vi "ToTable.vi"(8 "error in":errorcluster, 9 "Table Index (0)":i32, 10 "variant":variant, 11 "Benchmark PID editor node in":refnum<class "Benchmark PID editor node.lvclass">) -> (0 "error out":errorcluster, 1 "row headers":string[](array[string]), 2 "table":string[][](array[string]), 3 "Benchmark PID editor node out":refnum<class "Benchmark PID editor node.lvclass">)   [LabVIEW 2018, in "Benchmark PID editor node.lvclass"]
doc: "Generates the strings needed to display on a table based on the information found in the engine and module configuration classes."
uses:
  Benchmark PID editor node.lvclass
  module/configuration/Benchmark PID configuration.lvclass
  <vilib>/NI/Tag Bus/tag/tag descriptor.lvclass
  <vilib>/NI/Module Execution Interface/Engine Configuration/engine configuration.lvclass
  <vilib>/NI/Configuration Framework/serializable configuration/NISE_CEF_serializable configuration.lvclass
  C:/Program Files (x86)/National Instruments/LabVIEW 2018/vi.lib/NI/Tag Bus Module Framework/module configuration/TBM module configuration.lvclass
  C:/Program Files (x86)/National Instruments/LabVIEW 2018/vi.lib/NI/Tag Bus Module Framework/root configuration/TBM configuration.lvclass
  C:/Program Files (x86)/National Instruments/LabVIEW 2018/vi.lib/NI/Configuration Framework/serializable configuration/NISE_CEF_serializable configuration.lvclass
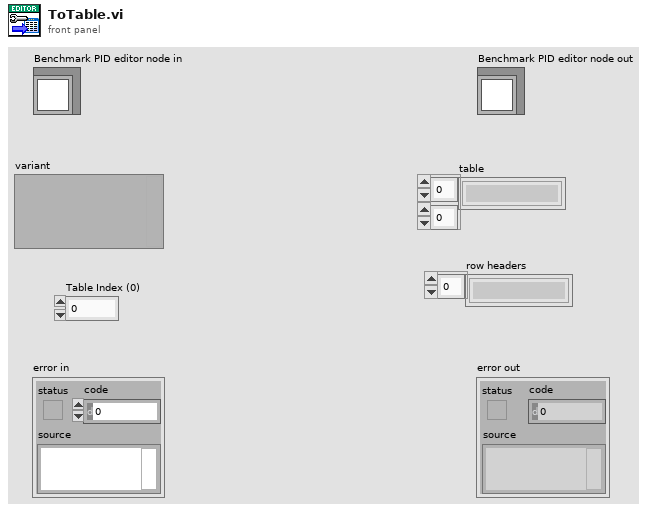
[diagram p1: front panel]
types:
  T1 = typedef "Benchmark PID configuration.lvclass/Line.ctl" = cluster{"PID Name":string, "Setpoint":refnum<class "TBM channel.lvclass">, "Variable":refnum<class "TBM channel.lvclass">, "Output":refnum<class "TBM channel.lvclass">}
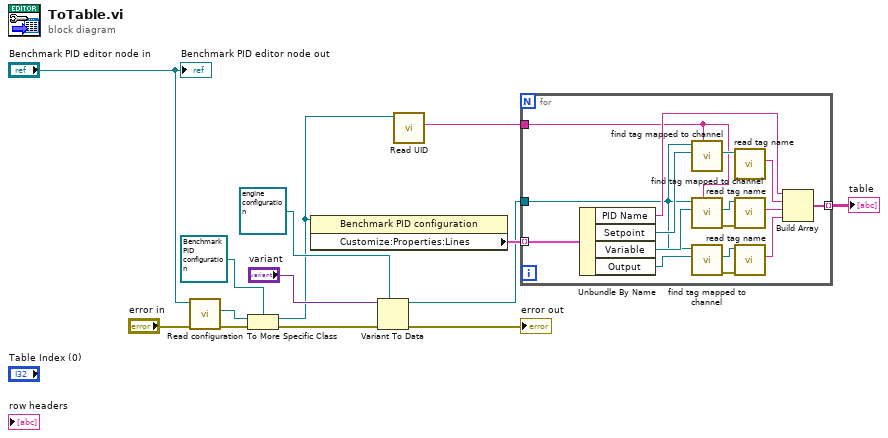
[diagram p0: block diagram]
diagram:
  n1 = call-dynamic "Read configuration.vi"("error in"="error in", "Benchmark PID editor node in"="Benchmark PID editor node in") -> ("error out"=w14:errorcluster, "configuration"=w5:refnum<class "NISE_CEF_serializable configuration.lvclass">)  [unwired: 7 in, 1 out]
  n2 = To More Specific Class(target class=refnum<class "Benchmark PID configuration.lvclass"> refnum ("tag bus configurable plugin module configuration"), reference=w5, error in=w14) -> (specific class reference=w4:refnum<class "Benchmark PID configuration.lvclass">, error out=w2:errorcluster)
  n3 = property class="Benchmark PID configuration"(reference=w4) -> ("Customize:Properties:Lines"=w11:T1[])  [unwired: 1 in, 2 out]
  n4 = Variant To Data(error in=w2, type=refnum<class "engine configuration.lvclass"> refnum ("engine configuration"), Variant="variant") -> (data=w8:refnum<class "engine configuration.lvclass">, error out=→"error out":errorcluster)
  n5 = call <vilib>:"Read UID.vi"("configuration in"=w4) -> ("instance id"=w3:string)  [unwired: 8 in, 2 out]
  n6 = for {
    tunnel: w11 -> [w30] mode=indexing
    tunnel: w8 -> [w17]
    tunnel: [w26] -> w6 mode=indexing
    tunnel: w3 -> [w21]
    n7 = Unbundle By Name(w30) -> ("PID Name"=w25:string, "Setpoint"=w27:refnum<class "TBM channel.lvclass">, "Variable"=w20:refnum<class "TBM channel.lvclass">, "Output"=w18:refnum<class "TBM channel.lvclass">)
    n8 = call <vilib>:"find tag mapped to channel.vi"("owner"=w21, "channel"=w27, "engine configuration in"=w17) -> ("tag"=w29:refnum<class "tag descriptor.lvclass">)  [unwired: 6 in, 2 out]
    n9 = call <vilib>:"find tag mapped to channel.vi"("owner"=w21, "channel"=w20, "engine configuration in"=w17) -> ("error out"=w24:errorcluster, "tag"=w23:refnum<class "tag descriptor.lvclass">)  [unwired: 6 in, 1 out]
    n10 = call <vilib>:"find tag mapped to channel.vi"("channel"=w18, "engine configuration in"=w17) -> ("error out"=w19:errorcluster, "tag"=w16:refnum<class "tag descriptor.lvclass">)  [unwired: 7 in, 1 out]
    n11 = call <vilib>:"read tag name.vi"("system tag in"=w29) -> ("name"=w28:string)  [unwired: 8 in, 2 out]
    n12 = call <vilib>:"read tag name.vi"("error in"=w24, "system tag in"=w23) -> ("name"=w22:string)  [unwired: 7 in, 2 out]
    n13 = call <vilib>:"read tag name.vi"("error in"=w19, "system tag in"=w16) -> ("name"=w15:string)  [unwired: 7 in, 2 out]
    n14 = Build Array(w25, w28, w22, w15) -> (w26:string[])
  }
  "table" <- w6
  "Benchmark PID editor node out" <- "Benchmark PID editor node in"
